vi "Setup subWorker - ScopeSim.vi"(8 "error in":errorcluster, 11 "Head_ScopeSim in":refnum<class "Head_ScopeSim.lvclass">) -> (0 "error out":errorcluster, 3 "Head_ScopeSim out":refnum<class "Head_ScopeSim.lvclass">)   [LabVIEW 2019, in "Head_ScopeSim.lvclass"]
doc: "This VI sets up the framework parameters of a statically-linked subWorker."
uses:
  Head_ScopeSim.lvclass
  Scope Simulator/Scope Simulator.lvclass
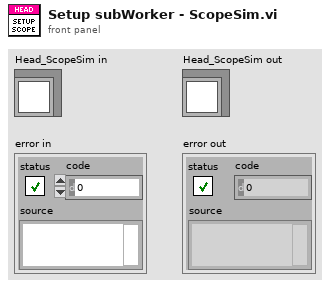
[diagram p1: front panel]
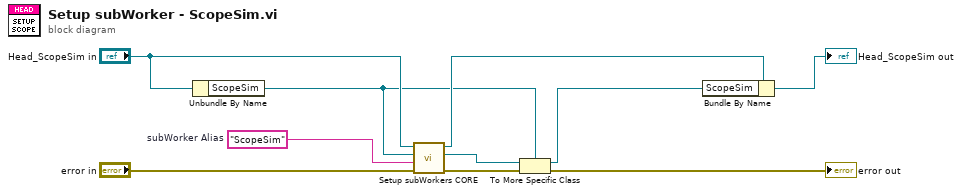
[diagram p0: block diagram]
diagram:
  w6 = "ScopeSim"  # subWorker Alias
  n1 = Unbundle By Name("Head_ScopeSim in") -> ("ScopeSim"=w3:refnum<class "Scope Simulator.lvclass">)
  n2 = call-dynamic "Setup subWorkers CORE.vi"("error in"="error in", "subWorker Alias"=w6, "subWorker"=w3, "Worker"="Head_ScopeSim in") -> ("error out"=w5:errorcluster, "subWorker out"=w1:refnum<class "Worker.lvclass">, "Worker out"=w8:refnum<class "Head_ScopeSim.lvclass">)  [unwired: 5 in]
  n3 = To More Specific Class(target class=w3, reference=w1, error in=w5) -> (specific class reference=w2:refnum<class "Scope Simulator.lvclass">, error out=→"error out":errorcluster)
  n4 = Bundle By Name(cluster=w8, "ScopeSim"=w2) -> (→"Head_ScopeSim out":refnum<class "Head_ScopeSim.lvclass">)
